vi "Do.vi"(8 "error in (no error)":errorcluster, 10 "Actor in":refnum<class "Actor.lvclass">, 11 "Update Msg in":refnum<class "Update Msg.lvclass">) -> (0 "error out":errorcluster, 2 "Actor out":refnum<class "Actor.lvclass">)   [LabVIEW 2016, in "Timed Loop Controller.lvlib" / "Update Msg.lvclass"]
doc: "This VI delivers the message to the actor by calling the appropriate method(s) on the actor."
uses:
  Update Msg.lvclass
  <vilib>/ActorFramework/Actor/Actor.lvclass
  Timed Loop Controller/Timed Loop Controller.lvclass
  C:/Program Files (x86)/National Instruments/LabVIEW 2016/vi.lib/ActorFramework/Actor/Actor.lvclass
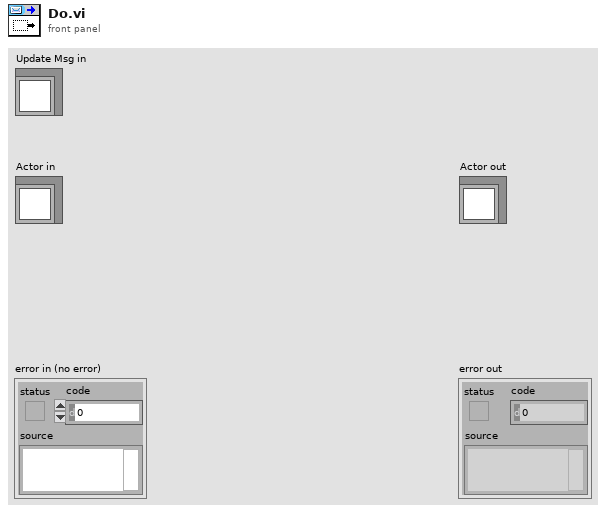
[diagram p1: front panel]
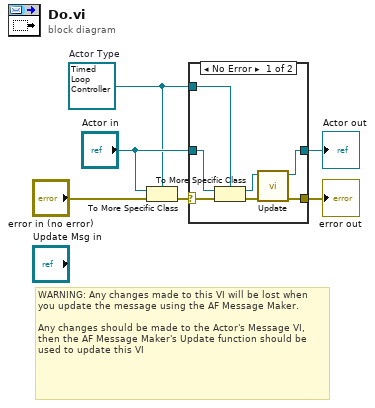
[diagram p0: block diagram]
diagram:
  w1 = refnum<class "Timed Loop Controller.lvclass"> refnum  # Actor Type
  # "WARNING: Any changes made to this VI will be lost when you update the message using the AF Message Maker.\n\nAny changes should be made to the Actor's Message VI, then the AF Message Maker's Update function should be used to update this VI"
  n1 = To More Specific Class(target class=w1, reference="Actor in", error in="error in (no error)") -> (error out=w5:errorcluster)  [unwired: 1 out]
  n2 = case shown="No Error" w5 {
    selector: w5 -> [w13 w15]
    tunnel: [w8 w15] -> w4
    tunnel: [w7 w14] -> w3
    tunnel: "Actor in" -> [w12 w14]
    tunnel: w1 -> [w11 _]
    frame No Error {
      n3 = To More Specific Class ("Actor Cast")(target class=w11, reference=w12, error in=w13) -> (specific class reference=w10:refnum<class "Timed Loop Controller.lvclass">, error out=w9:errorcluster)
      n4 = call-dynamic "Update.vi"("error in (no error)"=w9, "Timed Loop Controller in"=w10) -> ("error out"=w8:errorcluster, "Timed Loop Controller out"=w7:refnum<class "Timed Loop Controller.lvclass">)  [unwired: 8 in]
    }
    frame Error {
    }
  }
  "error out" <- w4
  "Actor out" <- w3
